vi "Check Initial Reply.vi"(7 "Write Message":u8[](array[numeric]), 8 "error in (no error)":errorcluster, 11 "Reply":T1[](array[typedef]) {"payload" format="%x"; "timestamp" format="%<%.7X\n%x>T"; "type" items=["CAN Data"=0, "CAN Remote"=1, "CAN Bus Error"=2, "J1939 Data"=192, "Delay"=224, "Log Trigger"=225, "Start Trigger"=226]; "identifier" format="%x"}) -> (0 "error out":errorcluster, 2 "Message Failed?  2":bool, 3 "Data Packet 2":u8[](array[numeric]), 5 "Whole Payload":u8[](array[numeric]))   [LabVIEW 2015, in "Oil.lvclass"]
uses:
  Oil.lvclass
  <vilib>/xnet/xnet.llb/XNET Frame CAN.ctl
  <vilib>/xnet/xnet.llb/XNET Frame Type CAN.ctl
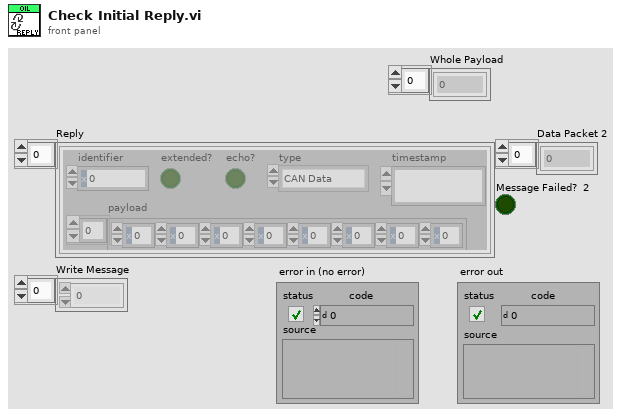
[diagram p1: front panel]
types:
  T1 = typedef "XNET Frame CAN.ctl" = cluster{"timestamp":timestamp, "payload":u8[], "identifier":u32, "type":T2, "extended?":bool, "echo?":bool}
  T2 = typedef "XNET Frame Type CAN.ctl" = u8
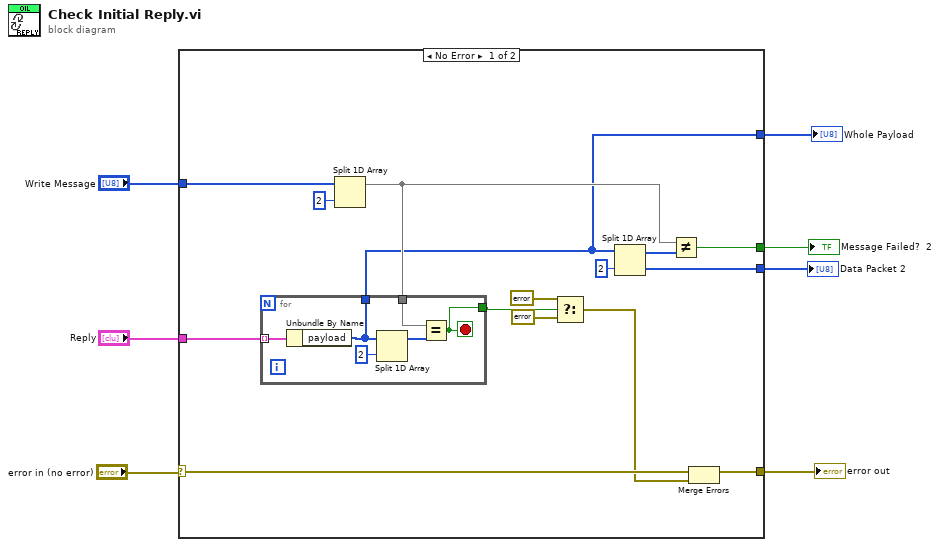
[diagram p0: block diagram]
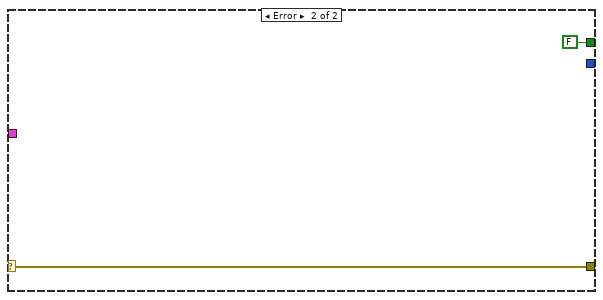
[diagram p2: hidden frame]
diagram:
  n1 = case shown="No Error" "error in (no error)" {
    selector: "error in (no error)" -> [w10 w30]
    tunnel: "Write Message" -> [w22 _]
    tunnel: [w18 _] -> w6
    tunnel: [w17 FALSE] -> w5
    tunnel: "Reply" -> [w16 _]
    tunnel: [w14 _] -> w3
    tunnel: [w8 w30] -> w1
    frame No Error {
      n2 = Split 1D Array(array=w22, index=2) -> (first subarray=w15:u8[])  [unwired: 1 out]
      n3 = for {
        tunnel: w16 -> [w28] mode=indexing
        tunnel: w15 -> [w25]
        tunnel: [w24] -> w14
        tunnel: [w23] -> w11
        stop <- w23 stop-if-true
        n4 = Unbundle By Name(w28) -> ("payload"=w24:u8[])
        n5 = Split 1D Array(array=w24, index=2) -> (first subarray=w26:u8[])  [unwired: 1 out]
        n6 = Equal?(x=w25, y=w26) -> (x = y?=w23:bool)
      }
      n7 = Select(t=errorcluster {"status"=FALSE, "code"=0, "source"=""} ("error in (no error)"), s=w11, f=errorcluster {"status"=TRUE, "code"=786, "source"="No response from intended CAN Board "} ("error in (no error)")) -> (s? t:f=w9:errorcluster)
      n8 = Split 1D Array(array=w14, index=2) -> (first subarray=w19:u8[], second subarray=w18:u8[])
      n9 = Not Equal?(x=w15, y=w19) -> (x != y?=w17:bool)
      n10 = Merge Errors(w10, w9) -> (w8:errorcluster)
    }
    frame Error {
    }
  }
  "Data Packet 2" <- w6
  "Message Failed?  2" <- w5
  "Whole Payload" <- w3
  "error out" <- w1
